vi "985x Properties.vi"() -> ()   [LabVIEW 2020, in "985x Support Addon Engine.lvlib"]
uses:
  985x Support Addon Engine.lvlib
panel:
  in  "Rx FIFO Name":string="985x_Rx_CAN"
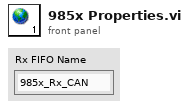
[diagram p1: front panel]
diagram:
